vi "Store Actors.vi"(8 "error in (no error)":errorcluster, 9 "Actor Paths":path[](array[path]), 10 "Actors":string[](array[string]), 11 "Target Store in":refnum<class "Live Store.lvclass">) -> (0 "error out":errorcluster, 3 "Target Store out":refnum<class "Live Store.lvclass">)   [LabVIEW 2023, in "Add Async Methods Actor.lvlib" / "Live Store.lvclass"]
uses:
  Live Store.lvclass
  Live Store.lvclass/Live Store.ctl
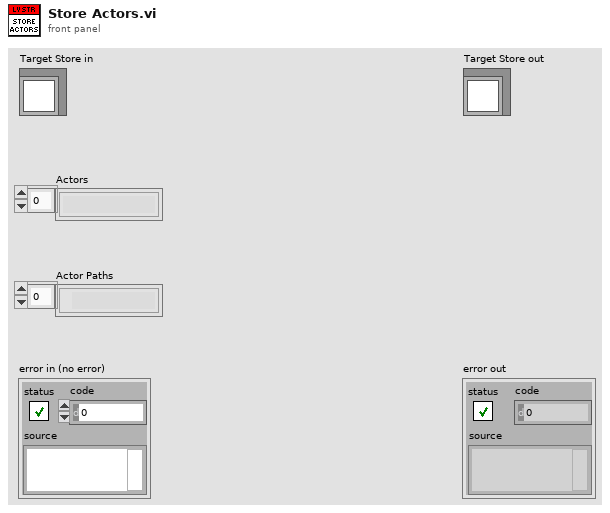
[diagram p1: front panel]
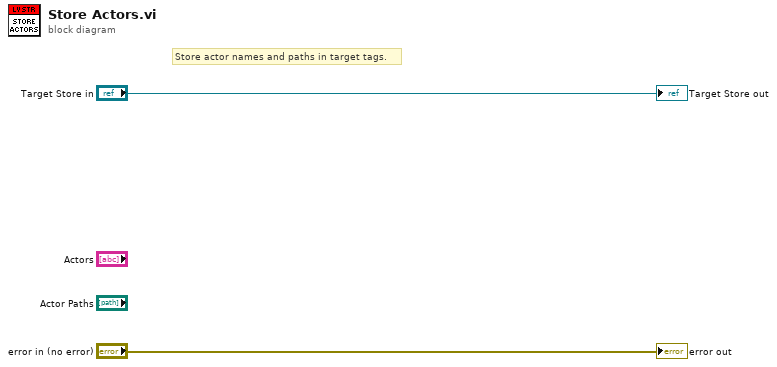
[diagram p0: block diagram]
diagram:
  # "Store actor names and paths in target tags."
  "error out" <- "error in (no error)"
  "Target Store out" <- "Target Store in"
